vi "Getter Scripting.vi"(10 "Accessor Options":T1, 11 "VI Refnum":refnum<vi>) -> ()   [LabVIEW 2018, in "LVClassByRef.lvlib"]
uses:
  <resource>/Framework/Providers/LVClassByRef/LVClassByRef.lvlib
  <resource>/Framework/Providers/LVClassByRef/Accessor Options.ctl
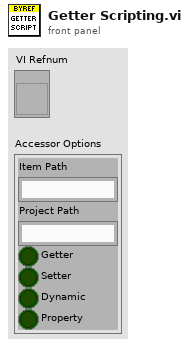
[diagram p1: front panel]
types:
  T1 = typedef "LVClassByRef.lvlib/Accessor Options.ctl" = cluster{"Item Path":string, "Project Path":string, "Getter":bool, "Setter":bool, "Dynamic":bool, "Property":bool}
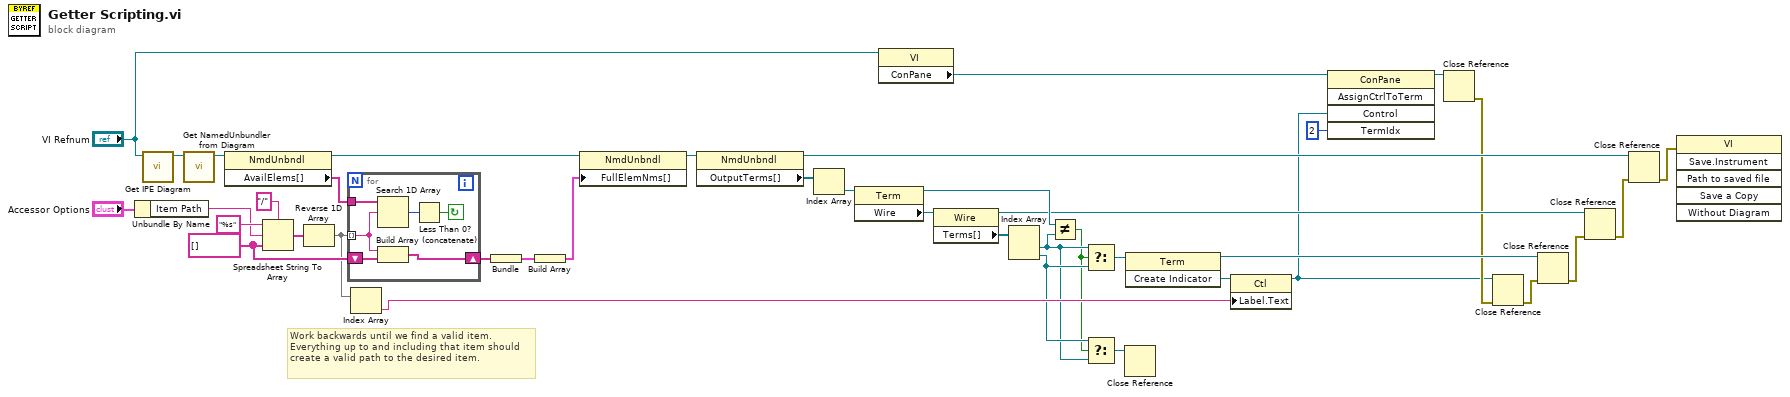
[diagram p0: block diagram]
diagram:
  w33 = string[] []
  # "Work backwards until we find a valid item. Everything up to and including that item should create a valid path to the desired item."
  n1 = Unbundle By Name("Accessor Options") -> ("Item Path"=w37:string)
  n2 = call <resource>:"Get IPE Diagram.vi"("VI Ref"="VI Refnum") -> ("IPE Diagram"=w36:refnum<vi>)  [unwired: 10 in]
  n3 = call <resource>:"Get NamedUnbundler from Diagram.vi"("Diagram"=w36) -> ("UBN Node"=w35:refnum<vi>)  [unwired: 10 in]
  n4 = property class="NmdUnbndl"(reference=w35) -> (reference out=w31:refnum<vi>, "AvailElems[]"=w32:string[])  [unwired: 1 in, 1 out]
  n5 = Spreadsheet String To Array(delimiter (Tab)="/", format string="%s", spreadsheet string=w37, array type (2D Dbl)=w33) -> (array=w34:string[])
  n6 = Reverse 1D Array(array=w34) -> (reversed array=w19:string[])
  n7 = for {
    tunnel: w19 -> [w43] mode=indexing
    tunnel: w32 -> [w46]
    shift-right: [w42] -> w30
    shift-left: w33 -> [w44]
    stop <- w41 continue-if-true
    n8 = Search 1D Array(1D array=w46, element=w43) -> (index of element=w45:i32)  [unwired: 1 in]
    n9 = Build Array (concatenate)(w43, w44) -> (w42:string[])
    n10 = Less Than 0?(x=w45) -> (x < 0?=w41:bool)
  }
  n11 = Index Array(array=w19) -> (element=w18:string)  [unwired: 1 in]
  n12 = Bundle(w30) -> (w29:cluster{string[]})  [unwired: 1 in]
  n13 = Build Array(w29) -> (w28:cluster{string[]}[])
  n14 = property class="NmdUnbndl"(reference=w31, "FullElemNms[]"=w28) -> (reference out=w27:refnum<vi>)  [unwired: 1 in, 1 out]
  n15 = property class="NmdUnbndl"(reference=w27) -> (reference out=w9:refnum<vi>, "OutputTerms[]"=w26:refnum<vi>[])  [unwired: 1 in, 1 out]
  n16 = Index Array(array=w26) -> (element=w25:refnum<vi>)  [unwired: 1 in]
  n17 = property class="Term"(reference=w25) -> (reference out=w22:refnum<vi>, "Wire"=w24:refnum<vi>)  [unwired: 1 in, 1 out]
  n18 = property class="VI"(reference="VI Refnum") -> ("ConPane"=w5:refnum<vi>)  [unwired: 1 in, 2 out]
  n19 = property class="Wire"(reference=w24) -> (reference out=w11:refnum<vi>, "Terms[]"=w23:refnum<vi>[])  [unwired: 1 in, 1 out]
  n20 = Index Array(array=w23) -> (element #1=w14:refnum<vi>, element #2=w15:refnum<vi>)  [unwired: 2 in]
  n21 = Not Equal?(x=w22, y=w14) -> (x != y?=w13:bool)
  n22 = Select(t=w14, s=w13, f=w15) -> (s? t:f=w21:refnum<vi>)
  n23 = Select(t=w15, s=w13, f=w14) -> (s? t:f=w12:refnum<vi>)
  n24 = Close Reference(reference=w12) -> ()  [unwired: 1 in, 1 out]
  n25 = invoke class="Term" method="Create Indicator"(reference=w21) -> (reference out=w17:refnum<vi>, "Create Indicator"=w20:refnum<vi>)  [unwired: 2 in, 1 out]
  n26 = property class="Ctl"(reference=w20, "Label.Text"=w18) -> (reference out=w1:refnum<vi>)  [unwired: 1 in, 1 out]
  n27 = invoke class="ConPane" method="AssignCtrlToTerm"(reference=w5, "Control"=w1, "TermIdx"=u32 2 ("Terminal Index")) -> (reference out=w3:refnum<vi>)  [unwired: 2 in, 4 out]
  n28 = Close Reference(reference=w3) -> (error out=w2:errorcluster)  [unwired: 1 in]
  n29 = Close Reference(reference=w1, error in (no error)=w2) -> (error out=w16:errorcluster)
  n30 = Close Reference(reference=w17, error in (no error)=w16) -> (error out=w10:errorcluster)
  n31 = Close Reference(reference=w11, error in (no error)=w10) -> (error out=w8:errorcluster)
  n32 = Close Reference(reference=w9, error in (no error)=w8) -> (error out=w7:errorcluster)
  n33 = invoke class="VI" method="Save.Instrument"(error in=w7) -> ()  [unwired: 5 in, 6 out]
